vi "Get Channel Data.vi"(9 "Digits of Precision":u32, 10 "Original T0":timestamp, 11 "waveform in":waveform(dbl)) -> (2 "Corrected Data":dbl[](array[numeric]), 3 "Resulting Data String":string[](array[string]))   [LabVIEW 2022 SP3, in "CSV Export.lvlib" / "CSV Export.lvclass"]
uses:
  CSV Export.lvclass
  CSV Export.lvclass/CSV Export.ctl
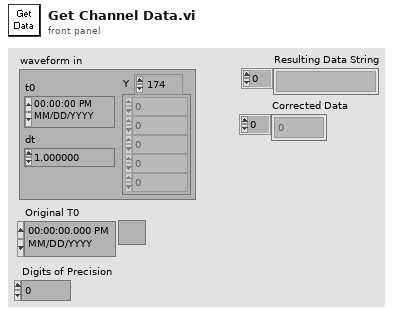
[diagram p1: front panel]
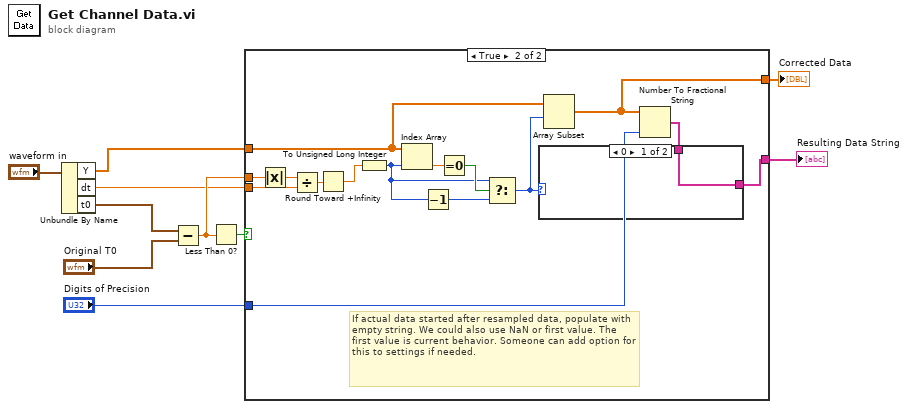
[diagram p0: block diagram]
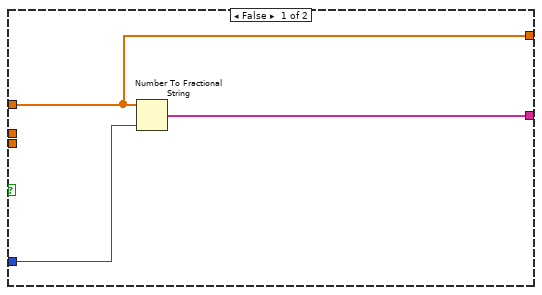
[diagram p2: hidden frame]
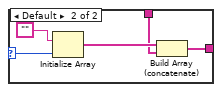
[diagram p3: hidden frame]
diagram:
  n1 = Unbundle By Name("waveform in") -> ("Y"=w4:dbl[], "dt"=w6:dbl, "t0"=w8:timestamp)
  n2 = Subtract(x=w8, y="Original T0") -> (x-y=w7:dbl)
  n3 = Less Than 0?(x=w7) -> (x < 0?=w5:bool)
  n4 = case shown="True" w5 {
    tunnel: w7 -> [_ w28]
    tunnel: w6 -> [_ w27]
    tunnel: w4 -> [w11 w19]
    tunnel: "Digits of Precision" -> [w13 w18]
    tunnel: [w12 w16] -> w2
    tunnel: [w11 w15] -> w1
    frame False {
      n5 = Number To Fractional String(number=w11, precision (6)=w13) -> (F-format string=w12:string[])  [unwired: 2 in]
    }
    frame True {
      # "If actual data started after resampled data, populate with empty string. We could also use NaN or first value. The first value is current behavior. Someone can add option for this to settings if needed."
      n6 = Absolute Value(x=w28) -> (abs(x)=w26:dbl)
      n7 = Divide(x=w26, y=w27) -> (x/y=w25:dbl)
      n8 = Round Toward +Infinity(x=w25) -> (ceil(x): smallest int >= x=w23:dbl)
      n9 = To Unsigned Long Integer(number=w23) -> (unsigned 32bit integer=w21:u32)
      n10 = Index Array(array=w19, index=w21) -> (element=w24:dbl)
      n11 = Decrement(x=w21) -> (x-1=w20:u32)
      n12 = Equal To 0?(x=w24) -> (x = 0?=w22:bool)
      n13 = Select(t=w21, s=w22, f=w20) -> (s? t:f=w14:u32)
      n14 = Array Subset(array=w19, index=w14) -> (w15:dbl[])  [unwired: 1 in]
      n15 = Number To Fractional String(number=w15, precision (6)=w18) -> (F-format string=w17:string[])  [unwired: 2 in]
      n16 = case shown="0" w14 {
        selector: w14 -> [_ w30]
        tunnel: w17 -> [w29 w32]
        tunnel: [w29 w31] -> w16
        frame 0 {
        }
        frame Default {
          n17 = Initialize Array("", w30) -> (w33:string[])
          n18 = Build Array (concatenate)(w33, w32) -> (w31:string[])
        }
      }
    }
  }
  "Resulting Data String" <- w2
  "Corrected Data" <- w1
